vi "State(FGV).vi"(8 "Error In":errorcluster, 9 "Action":enum16{"Set", "Get"}(ring), 11 "input state":T2) -> (0 "Error Out":errorcluster, 2 "Output \nIndicator":T1 caption="Z     Y     X", 3 "output state":T2)   [LabVIEW 2023]
doc: "This VI realizes a functional global variable that stores the current state of the FSM."
uses:
  controls/enum defining states.ctl
  controls/Boolean output indicator.ctl
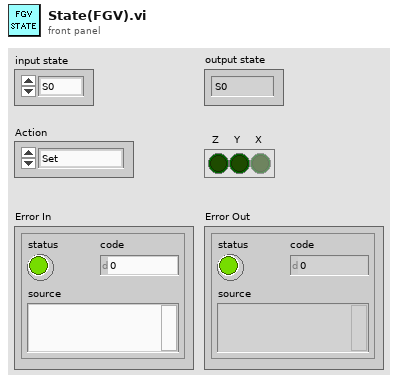
[diagram p1: front panel]
types:
  T1 = typedef "Boolean output indicator.ctl" = bool[]
  T2 = typedef "enum defining states.ctl" = enum16{"S0", "S1", "S2", "S3"}
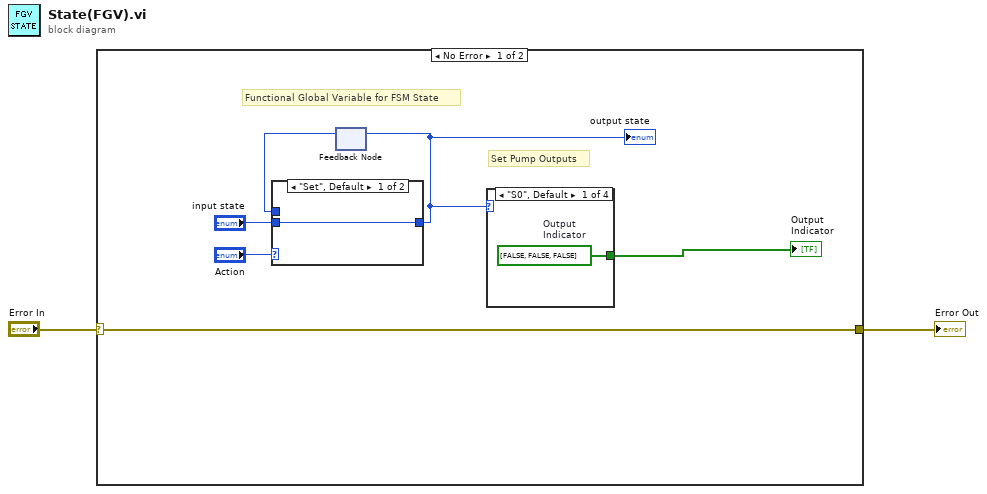
[diagram p0: block diagram]
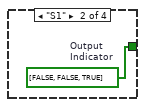
[diagram p2: hidden frame]
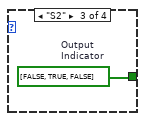
[diagram p3: hidden frame]
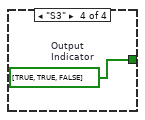
[diagram p4: hidden frame]
diagram:
  n1 = case shown="No Error" "Error In" {
    selector: "Error In" -> [w7 w15]
    tunnel: [w7 w15] -> w1
    frame No Error {
      # "Set Pump Outputs"
      # "Functional Global Variable for FSM State"
      n2 = feedback #1() -> (w4:T2)  [unwired: 1 in]
      n3 = case shown="\"Set\", Default" "Action" {
        tunnel: "input state" -> [w13 _]
        tunnel: [w13 w14] -> w3
        tunnel: w4 -> [_ w14]
        frame "Set", Default {
        }
        frame "Get" {
        }
      }
      "output state" <- w3
      n4 = feedback-in #1(w3) -> ()
      n5 = case shown="\"S0\", Default" w3 {
        tunnel: [w9 w10 w11 w12] -> w5
        frame "S0", Default {
          w9 = T1 [FALSE, FALSE, FALSE]  # Output  Indicator
        }
        frame "S1" {
          w10 = T1 [FALSE, FALSE, TRUE]  # Output  Indicator
        }
        frame "S2" {
          w11 = T1 [FALSE, TRUE, FALSE]  # Output  Indicator
        }
        frame "S3" {
          w12 = T1 [TRUE, TRUE, FALSE]  # Output  Indicator
        }
      }
      "Output \nIndicator" <- w5
    }
    frame Error {
    }
  }
  "Error Out" <- w1
